vi "fpga_trigger_test.vi"() -> ()   [LabVIEW 2014]
uses:
  <instrlib>/_niInstr/Streaming/v1/Common/Stream State.ctl
  <vilib>/Platform/TimedLoop/XDataNode/timing_clust.ctl
  <vilib>/Platform/TimedLoop/XDataNode/nitl_modes.ctl
  <vilib>/Platform/TimedLoop/XDataNode/wakeup.ctl
  <vilib>/rvi/Emulation/niFpgaSctlEmulationGetInTimedLoop.vi
  <vilib>/rvi/Emulation/niFpgaEmulationReportErrorSimple.vi
  <vilib>/rvi/Emulation/niFpgaGetClockAttributes.vi
  <vilib>/rvi/Emulation/niFpgaCriticalErrorInLSC.vi
  <vilib>/rvi/eio/common/nirviEmuTemplateMethod_errors.vi
  <instrlib>/_niInstr/Basic Elements/v1/FPGA/Private/Count Up U64.vi
  <vilib>/Platform/TimedLoop/XDataNode/XDataNode.xnode
  <vilib>/eio/EIONode/EIONode.xnode
  <instrlib>/_niInstr/Streaming/v1/FPGA/niInstr Streaming v1 FPGA.lvlib
  <instrlib>/_niInstr/Basic Elements/v1/FPGA/niInstr Basic Elements v1 FPGA.lvlib
  <vilib>/Platform/TimedLoop/XDataNode/XDNodeRunTimeDep.lvlib
  <instrlib>/_niInstr/Streaming/v1/Common/niInstr Streaming v1 Common.lvlib
panel:
  out "count out":u64
  out "out":bool
  out "request data":bool
  out "send data":bool
  in  "manual\ntrigger":bool
  in  "trigger \ndelay":u64
  in  "Clear Trigger":bool
  in  "stream.request state 0":T1
  in  "stream.num samples 0":u64
  out "stream.metadata 0":u64
  out "stream.samples transferred 0":u64
  out "stream.state 0":T1
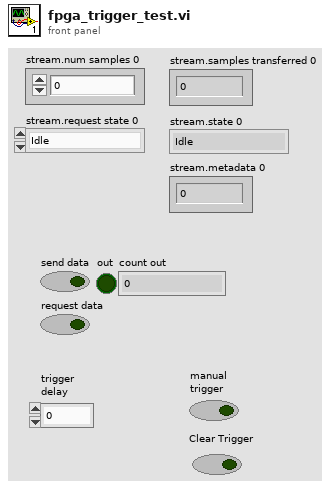
[diagram p1: front panel]
types:
  T1 = typedef "niInstr Streaming v1 Common.lvlib/Stream State.ctl" = enum8{"Idle", "Finite Transfer", "Continuous", "Done", "Error", "Not Ready", "Cancel"}
  T2 = typedef "XDNodeRunTimeDep.lvlib/timing_clust.ctl" = cluster{"Expected End [f-1]":u64, "Actual End [f-1]":u64, "Finished Late? [f-1]":bool, "Expected End [i-1]":u64, "Actual End [i-1]":u64, "Finished Late? [i-1]":bool, "Expected Start [i]":u64, "Actual Start [i]":u64, "Expected Start [f]":u64, "Actual Start [f]":u64, "Source Name":string, "Structure Name":string, "Period":i64, "Deadline":i64, "Offset":i64, "Start":i64, "Priority":i32, "Timeout":i32, "Mode":T3, "Wakeup Reason":T4, "Error":errorcluster, "Source Type":string, "Secondary Source Type":string, "Global End Time":u64, "Global Start Time":u64, "Frame Duration":u64, "Iteration Duration":u64, "Assigned CPU":i32, "I/O Scan Engine Mode":u32}
  T3 = typedef "XDNodeRunTimeDep.lvlib/nitl_modes.ctl" = enum32{"No Change", "Process missed periods, maintain original phase", "Discard missed periods, maintain original phase", "Process missed periods, ignore original phase", "Discard missed periods, ignore original phase"}
  T4 = typedef "XDNodeRunTimeDep.lvlib/wakeup.ctl" = enum32{"Normal", "Aborted", "Asynchronous wakeup", "Timing source error", "Timed loop error", "Timeout"}
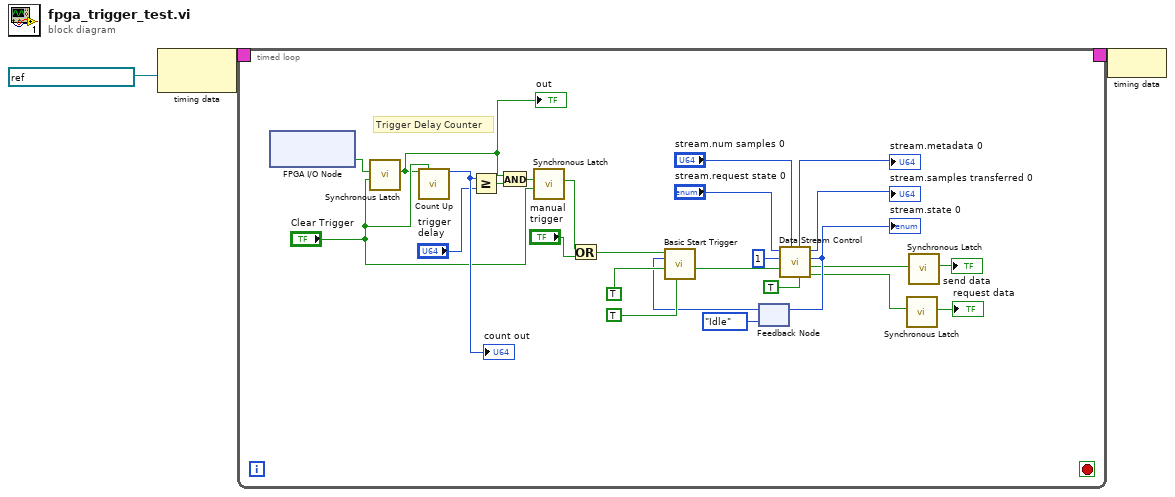
[diagram p0: block diagram]
diagram:
  n1 = node-c288(refnum<k21> "IO Module Clock 0" ("Source Name")) -> (w3:T2)
  n2 = timed-loop {
    timing: w3 -> [_]
    timing-out: [_] -> w2
    stop <- _ stop-if-true
    # "Trigger Delay Counter"
    n3 = xnode "FPGA I/O Node"() -> ("PXI_Star"=w22:bool)  [unwired: 1 in, 1 out]
    n4 = call <instrlib>:"Synchronous Latch.vi"("clear"="Clear Trigger", "set"=w22) -> ("out"=w16:bool)  [unwired: 9 in]
    "out" <- w16
    n5 = call-poly <instrlib>:"Count Up.vi"("increment"=w16, "reset"="Clear Trigger") -> ("count out"=w21:u64)  [unwired: 13 in]
    "count out" <- w21
    n6 = Greater Or Equal?(x=w21, y="trigger \ndelay") -> (x >= y?=w17:bool)
    n7 = And(x=w16, y=w17) -> (x .and. y?=w15:bool)
    n8 = call <instrlib>:"Synchronous Latch.vi"("clear"="Clear Trigger", "set"=w15) -> ("out"=w14:bool)  [unwired: 9 in]
    n9 = Or(x=w14, y="manual\ntrigger") -> (x .or. y?=w12:bool)
    n10 = feedback #1(Stream_State."Idle" ("stream.state 0")) -> (w10:T1)
    n11 = call <instrlib>:"Basic Start Trigger.vi"("ready for start trigger"=TRUE, "data valid?"=TRUE, "stream.state"=w10, "start trigger"=w12) -> ("data valid"=w19:bool)  [unwired: 7 in]
    n12 = call <instrlib>:"Data Stream Control.vi"("ready for input?"=TRUE, "stream.num samples 0"="stream.num samples 0", "data valid"=w19, "element count"=u16 1, "stream.request state 0"="stream.request state 0") -> ("request data"=w4:bool, "send data"=w7:bool, "stream.state 0"=w9:T1, "stream.samples transferred 0"=→"stream.samples transferred 0":u64, "stream.metadata 0"=→"stream.metadata 0":u64)  [unwired: 2 in]
    "stream.state 0" <- w9
    n13 = feedback-in #1(w9) -> ()
    n14 = call <instrlib>:"Synchronous Latch.vi"("set"=w4) -> ("out"=→"request data":bool)  [unwired: 10 in]
    n15 = call <instrlib>:"Synchronous Latch.vi"("set"=w7) -> ("out"=→"send data":bool)  [unwired: 10 in]
  }
  n16 = node-c288(w2) -> ()
